vi "Delete.vi"(8 "error in (no error)":errorcluster, 11 "Child Class in":refnum<class "Example Application.lvclass">) -> (0 "error out":errorcluster, 3 "Child Class out":refnum<class "Example Application.lvclass">)   [LabVIEW 2015, in "Example Application.lvlib" / "Example Application.lvclass"]
uses:
  Example Application.lvclass
  Example Application.lvclass/Example Application.ctl
  Properties/Example App Properties.lvclass
  CBTF Modules/Classes/Application/Class/Application.lvclass
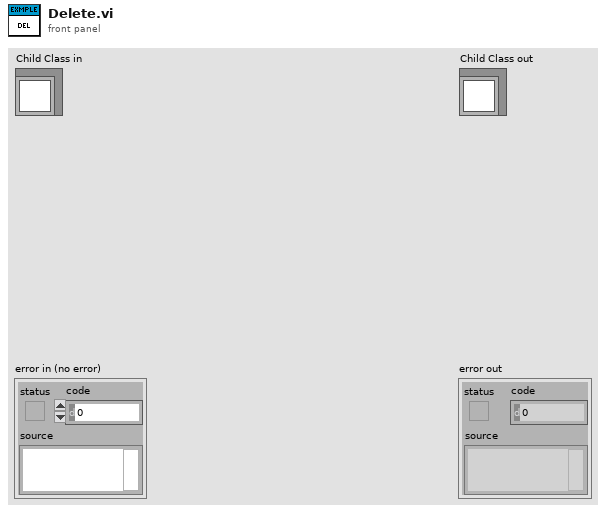
[diagram p1: front panel]
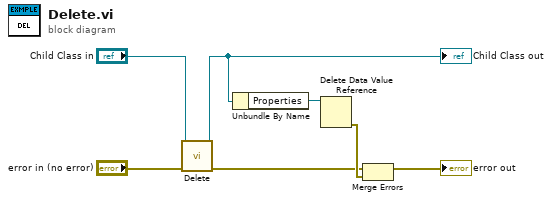
[diagram p0: block diagram]
diagram:
  n1 = call-parent "Delete.vi"("error in (no error)"="error in (no error)", "Child Class in"="Child Class in") -> ("error out"=w2:errorcluster, "Child Class out"=w3:refnum<class "Example Application.lvclass">)  [unwired: 8 in]
  "Child Class out" <- w3
  n2 = Unbundle By Name(w3) -> ("Properties"=w4:refnum<data-value>)
  n3 = Delete Data Value Reference(data value reference=w4) -> (error out=w5:errorcluster)  [unwired: 1 in, 1 out]
  n4 = Merge Errors(w2, w5) -> (→"error out":errorcluster)
